vi "Source V2.vi"(8 "error in":errorcluster, 9 "V2 rate":dbl=10.0, 10 "V2":dbl, 11 "VISA in":refnum<visa-resource-name>) -> (0 "error out":errorcluster, 1 "read buffer":string, 2 "format string":string="SOUR2:VOLT %3f.4:SLEW %3f.4", 3 "VISA out":refnum<visa-resource-name>)   [LabVIEW 2016]
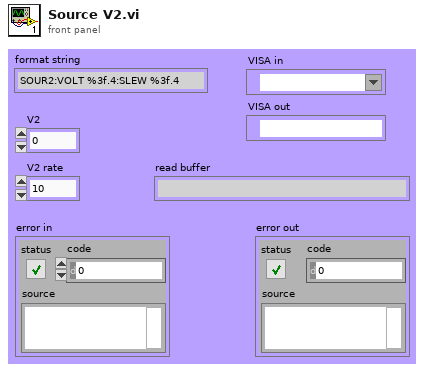
[diagram p1: front panel]
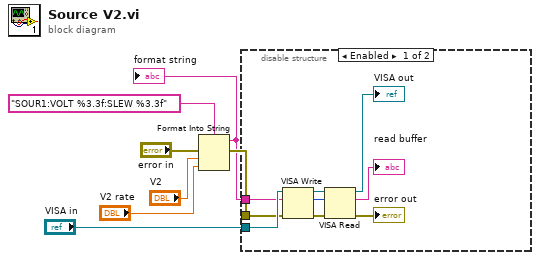
[diagram p0: block diagram]
diagram:
  n1 = Format Into String(format string="SOUR1:VOLT %3.3f:SLEW %3.3f", error in="error in", "V2", "V2 rate") -> (resulting string=w3:string, error out=w5:errorcluster)  [unwired: 1 in]
  "format string" <- w3
  n2 = disable-structure shown="Enabled" {
    disable-tunnel: "VISA in" -> [w16 _]
    disable-tunnel: w3 -> [w11 _]
    disable-tunnel: w5 -> [w10 _]
    frame Enabled {
      n3 = VISA Write(VISA resource name=w16, write buffer=w11, error in (no error)=w10) -> (VISA resource name out=w15:refnum<visa-resource-name>, return count=w14:u32, error out=w12:errorcluster)
      n4 = VISA Read(VISA resource name=w15, byte count=w14, error in (no error)=w12) -> (VISA resource name out=→"VISA out":refnum<visa-resource-name>, read buffer=→"read buffer":string, error out=→"error out":errorcluster)  [unwired: 1 out]
    }
    frame Disabled {
    }
  }
